vi "Convert number to decimal string and pad left with zeroes.vi"(10 "Width":u32, 11 "number":i32) -> (3 "result string":string)   [LabVIEW 2013]
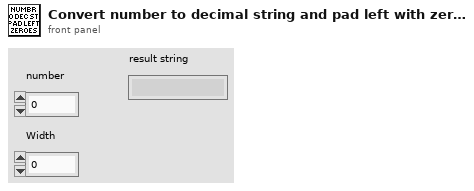
[diagram p1: front panel]
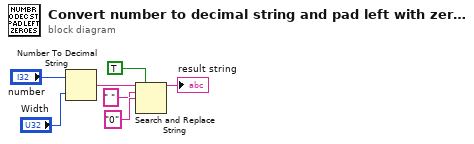
[diagram p0: block diagram]
diagram:
  n1 = Number To Decimal String(number="number", width (-)="Width") -> (decimal integer string=w1:string)
  n2 = Search and Replace String(replace all?=TRUE ("replace all? (F)"), input string=w1, search string=" ", replace string="0" ("replace string (\"\")")) -> (result string=→"result string":string)  [unwired: 4 in, 3 out]
